vi "State_Detect_Changes.vi"(7 "New state?":bool=TRUE, 8 "Old valves":bool[][](array[boolean]), 9 "New valves":bool[][](array[boolean]), 10 "Old flows":dbl[][](array[numeric]), 11 "New flows":dbl[][](array[numeric])) -> (2 "Values have changed":bool)   [LabVIEW 2025]
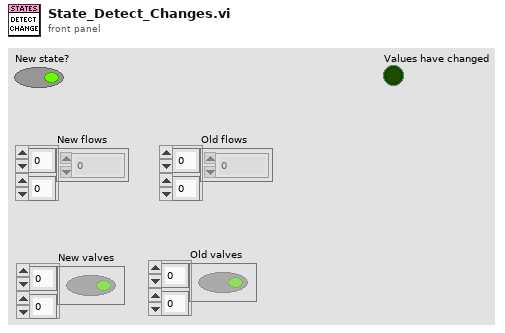
[diagram p1: front panel]
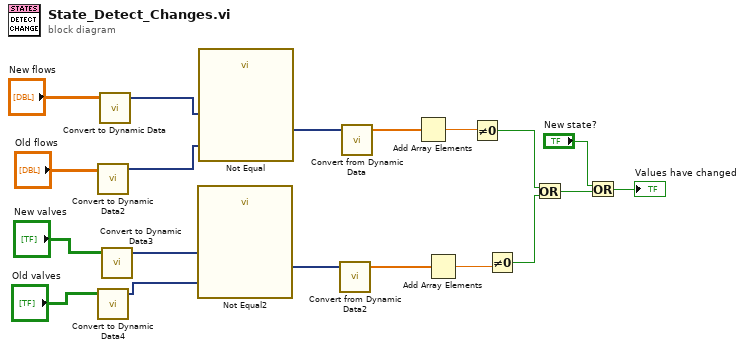
[diagram p0: block diagram]
diagram:
  n1 = call "Convert to Dynamic Data2"("2D Array"="Old flows") -> ("Dynamic Data Type"=w16:dynamicdata)  [unwired: 3 in]
  n2 = call "Convert to Dynamic Data4"("2D"="Old valves") -> ("Dynamic Data Type"=w11:dynamicdata)  [unwired: 3 in]
  n3 = call "Convert to Dynamic Data"("2D Array"="New flows") -> ("Dynamic Data Type"=w18:dynamicdata)  [unwired: 3 in]
  n4 = call "Convert to Dynamic Data3"("2D"="New valves") -> ("Dynamic Data Type"=w13:dynamicdata)  [unwired: 3 in]
  n5 = call "Not Equal2"("Operand 2"=w11, "Operand 1"=w13) -> ("Result"=w10:dynamicdata)  [unwired: 8 in, 1 out]
  n6 = call "Not Equal"("Operand 2"=w16, "Operand 1"=w18) -> ("Result"=w15:dynamicdata)  [unwired: 8 in, 1 out]
  n7 = call "Convert from Dynamic Data2"("Dynamic Data Type"=w10) -> ("Array"=w8:dbl[])  [unwired: 3 in]
  n8 = call "Convert from Dynamic Data"("Dynamic Data Type"=w15) -> ("Array"=w9:dbl[])  [unwired: 3 in]
  n9 = Add Array Elements(numeric array=w9) -> (sum=w7:dbl)
  n10 = Add Array Elements(numeric array=w8) -> (sum=w6:dbl)
  n11 = Not Equal To 0?(x=w7) -> (x != 0?=w5:bool)
  n12 = Not Equal To 0?(x=w6) -> (x != 0?=w4:bool)
  n13 = Or(x=w5, y=w4) -> (x .or. y?=w3:bool)
  n14 = Or(x="New state?", y=w3) -> (x .or. y?=→"Values have changed":bool)
